vi "Set Trajectory Mode.vi"(4 "Trajectory Mode":T1(ring), 5 "error in (no error)":errorcluster, 7 "Axis (1)":i32=1 min=1 max=3, 8 "VISA resource name":refnum<visa-resource-name>) -> (0 "error out":errorcluster, 3 "VISA resource name out":refnum<visa-resource-name>)   [LabVIEW 2015, in "Newport ESP301.lvlib"]
doc: "This command sets the <B>trajectory mode</B> on the axis specified by <B>Axis (1)</B>.\nChanging trajectory during motion is not allowed. Change trajectory mode only when the axis is not moving.\nIf the requested axis is member of a group, the controller returns error xx31, “COMMAND NOT ALLOWED DUE TO GROUP ASSIGNMENT”.\nFor a detailed description of motion profiles see the Motion Control Tutorial section (ESP301 User's manual)."
uses:
  <userlib>/Newport ESP301/Newport ESP301.lvlib
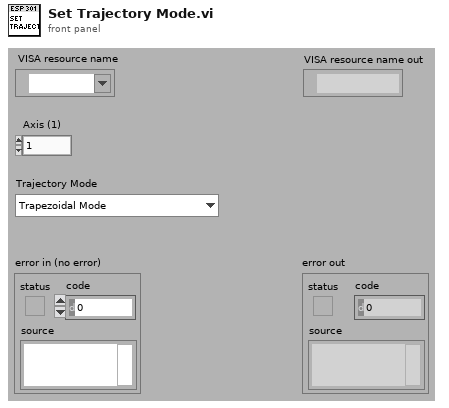
[diagram p1: front panel]
types:
  T1 = enum16{"Trapezoidal Mode", "S-curve Mode", "Jog Mode", "Slave to master's desired position (trajectory)", "Slave to master's actual position (feedback)", "Slave to master's actual velocity for jogging"}
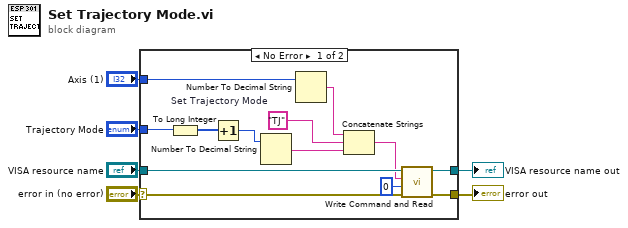
[diagram p0: block diagram]
diagram:
  n1 = case shown="No Error" "error in (no error)" {
    selector: "error in (no error)" -> [w18 w21]
    tunnel: [w17 w21] -> w5
    tunnel: "VISA resource name" -> [w19 w20]
    tunnel: [w16 w20] -> w3
    tunnel: "Axis (1)" -> [w12 _]
    tunnel: "Trajectory Mode" -> [w9 _]
    frame No Error {
      w14 = "TJ"  # Set Trajectory Mode
      n2 = To Long Integer(number=w9) -> (32bit integer=w8:i32)
      n3 = Increment(x=w8) -> (x+1=w7:i32)
      n4 = Number To Decimal String(number=w7) -> (decimal integer string=w15:string)  [unwired: 1 in]
      n5 = Number To Decimal String(number=w12) -> (decimal integer string=w13:string)  [unwired: 1 in]
      n6 = Concatenate Strings(w13, w14, w15) -> (w11:string)
      n7 = call <userlib>:"Write Command and Read.vi"("error in (no error)"=w18, "Bytes to read (100)"=u32 0, "Command"=w11, "VISA resource name"=w19) -> ("error out"=w17:errorcluster, "VISA resource name out"=w16:refnum<visa-resource-name>)  [unwired: 3 in, 1 out]
    }
    frame Error {
    }
  }
  "error out" <- w5
  "VISA resource name out" <- w3
